vi "SaveDataPathBuilder.vi"(10 "DataTypeSuffix":string, 11 "Inst name":string) -> (3 "Path name Out":path)   [LabVIEW 2018]
uses:
  Globals/Meas_global.vi
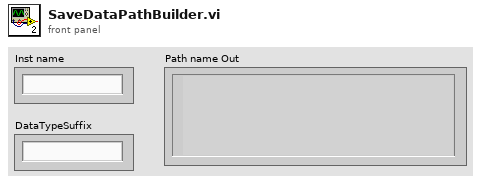
[diagram p1: front panel]
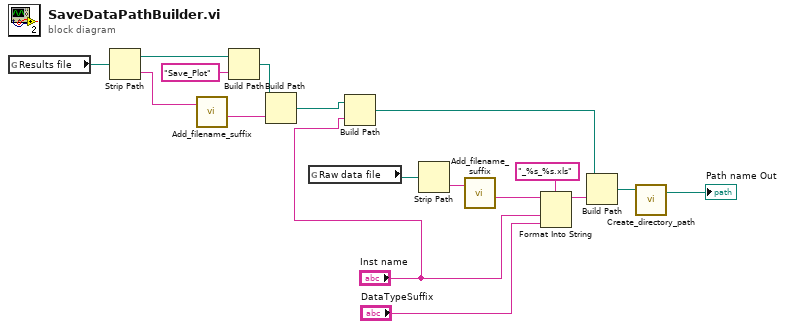
[diagram p0: block diagram]
diagram:
  n1 = global read "Meas_global.vi" "Results file"() -> (w4:path)
  n2 = Strip Path(path=w4) -> (stripped path=w7:path, name=w5:string)
  n3 = call "Add_filename_suffix.vi"("Filename"=w5) -> ("Base name"=w6:string)  [unwired: 1 in, 3 out]
  n4 = Build Path(base path=w7, name or relative path="Save_Plot") -> (appended path=w9:path)
  n5 = Build Path(base path=w9, name or relative path=w6) -> (appended path=w3:path)
  n6 = global read "Meas_global.vi" "Raw data file"() -> (w12:path)
  n7 = Build Path(base path=w3, name or relative path="Inst name") -> (appended path=w1:path)
  n8 = Strip Path(path=w12) -> (name=w10:string)  [unwired: 1 out]
  n9 = call "Add_filename_suffix.vi"("Filename"=w10) -> ("Base name"=w13:string)  [unwired: 1 in, 3 out]
  n10 = Format Into String(format string="_%s_%s.xls", initial string=w13, "Inst name", "DataTypeSuffix") -> (resulting string=w14:string)  [unwired: 1 in, 1 out]
  n11 = Build Path(base path=w1, name or relative path=w14) -> (appended path=w16:path)
  n12 = call "Create_directory_path.vi"("Path name"=w16) -> ("Path name Out"=→"Path name Out":path)  [unwired: 2 in, 1 out]
